vi "Open Log.vi"(8 "error in (no error)":errorcluster, 11 "Trace Controller in":refnum<class "Trace Controller.lvclass">) -> (0 "error out":errorcluster, 3 "Trace Controller out":refnum<class "Trace Controller.lvclass">)   [LabVIEW 2014, in "Robot Actor Framework.lvlib" / "Trace.lvlib" / "Trace Controller.lvclass"]
uses:
  Trace Controller.lvclass
  Trace Controller.lvclass/Trace Controller.ctl
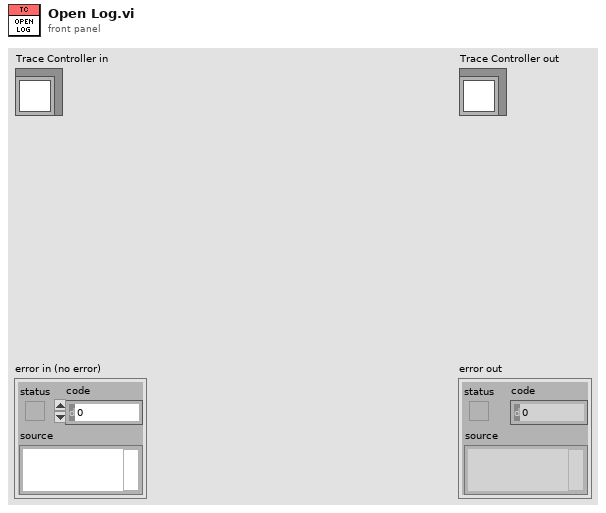
[diagram p1: front panel]
types:
  T1 = enum16{"open", "replace", "create", "open or create", "replace or create", "replace or create with confirmation"}
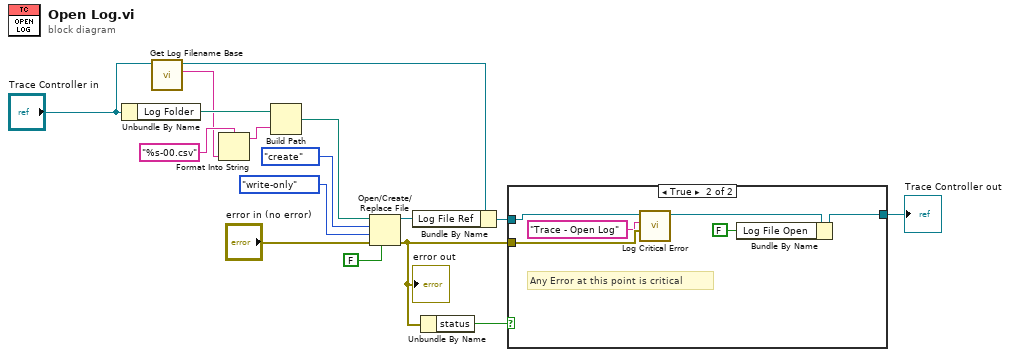
[diagram p0: block diagram]
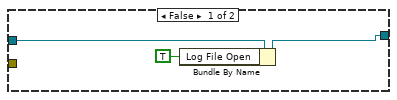
[diagram p2: hidden frame]
diagram:
  n1 = Unbundle By Name("Trace Controller in") -> ("Log Folder"=w16:path)
  n2 = call-dynamic "Get Log Filename Base.vi"("Trace Controller in"="Trace Controller in") -> ("Log Filename Base"=w8:string, "Trace Controller out"=w1:refnum<class "Trace Controller.lvclass">)  [unwired: 8 in, 1 out]
  n3 = Format Into String(format string="%s-00.csv", w8) -> (resulting string=w7:string)  [unwired: 2 in, 1 out]
  n4 = Build Path(base path=w16, name or relative path=w7) -> (appended path=w15:path)
  n5 = Open/Create/Replace File(file path (use dialog)=w15, error in="error in (no error)", operation (0:open)=T1."create", access (0:read/write)=enum16{"read/write", "read-only", "write-only"}."write-only", disable buffering (F)=FALSE) -> (refnum out=w11:refnum<file>, error out=w3:errorcluster)  [unwired: 1 in, 1 out]
  "error out" <- w3
  n6 = Bundle By Name(cluster=w1, "Log File Ref"=w11) -> (w5:refnum<class "Trace Controller.lvclass">)
  n7 = Unbundle By Name(w3) -> ("status"=w6:bool)
  n8 = case shown="True" w6 {
    tunnel: w5 -> [w19 w25]
    tunnel: [w18 w21] -> w4
    tunnel: w3 -> [_ w23]
    frame False {
      n9 = Bundle By Name(cluster=w19, "Log File Open"=TRUE) -> (w18:refnum<class "Trace Controller.lvclass">)
    }
    frame True {
      # "Any Error at this point is critical"
      n10 = call-dynamic "Log Critical Error.vi"("Critical Error"=w23, "Critical Error Event"="Trace - Open Log", "Trace Controller in"=w25) -> ("Trace Controller out"=w24:refnum<class "Trace Controller.lvclass">)  [unwired: 7 in, 1 out]
      n11 = Bundle By Name(cluster=w24, "Log File Open"=FALSE) -> (w21:refnum<class "Trace Controller.lvclass">)
    }
  }
  "Trace Controller out" <- w4
